vi "simpelkvant.vi"() -> ()   [LabVIEW 2013]
uses:
  <vilib>/DAQmx/write.llb/DAQmx Write (Digital 1D Bool NChan 1Samp 1Line).vi
  <vilib>/DAQmx/miscellaneous.llb/DAQmx Fill In Error Info.vi
panel:
  out "x+y":dbl
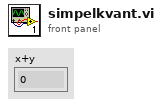
[diagram p1: front panel]
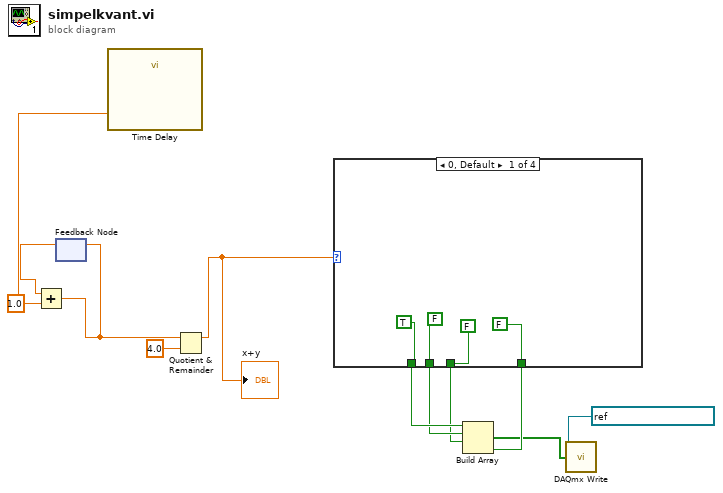
[diagram p0: block diagram]
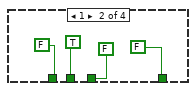
[diagram p2: hidden frame]
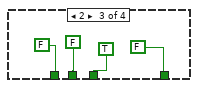
[diagram p3: hidden frame]
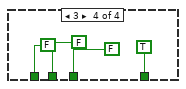
[diagram p4: hidden frame]
diagram:
  w10 = 1.0 ("y")
  n1 = feedback #1() -> (w11:dbl)  [unwired: 1 in]
  n2 = Add(x=w11, y=w10) -> (x+y=w9:dbl)
  n3 = feedback-in #1(w9) -> ()
  n4 = call "Time Delay"("Delay Time (s)"=w10) -> ()  [unwired: 10 in, 1 out]
  n5 = Quotient & Remainder(x=w9, y=4.0) -> (x-y*floor(x/y)=w7:dbl)  [unwired: 1 out]
  "x+y" <- w7
  n6 = case shown="0, Default" w7 {
    tunnel: [TRUE FALSE FALSE FALSE] -> w5
    tunnel: [FALSE TRUE FALSE FALSE] -> w4
    tunnel: [FALSE FALSE TRUE FALSE] -> w3
    tunnel: [FALSE FALSE FALSE TRUE] -> w2
    frame 0, Default {
    }
    frame 1 {
    }
    frame 2 {
    }
    frame 3 {
    }
  }
  n7 = Build Array(w5, w4, w3, w2) -> (w1:bool[])
  n8 = call-poly <vilib>:"DAQmx Write.vi"("task/channels in"=refnum<k21> "MyDigitalOutTask", "data"=w1) -> ()  [unwired: 11 in, 3 out]
